vi "4.7.vi"() -> ()   [LabVIEW 2017]
panel:
  out "猜测次数":i32
  out "随机数":i32
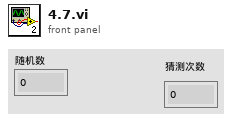
[diagram p1: front panel]
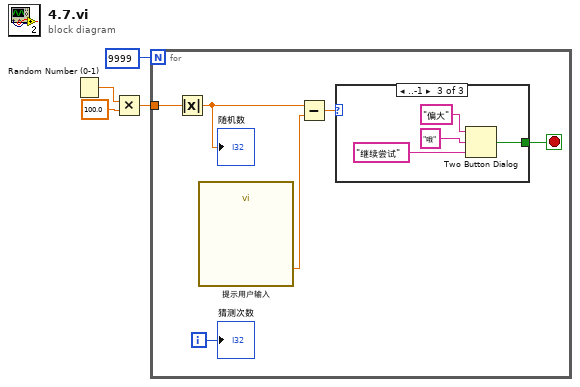
[diagram p0: block diagram]
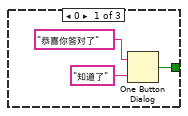
[diagram p2: hidden frame]
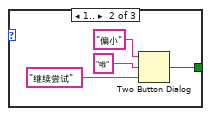
[diagram p3: hidden frame]
diagram:
  n1 = Random Number (0-1)() -> (number: 0 to 1=w2:dbl)
  n2 = Multiply(x=w2, y=100.0) -> (x*y=w3:dbl)
  n3 = for {
    N: 9999 -> [_]
    tunnel: w3 -> [w5]
    i -> [w8]
    stop <- w7 stop-if-true
    n4 = Absolute Value(x=w5) -> (abs(x)=w10:dbl)
    "随机数" <- w10
    n5 = call "提示用户输入"() -> ("请在1-1000猜"=w6:dbl)  [unwired: 17 in, 2 out]
    n6 = Subtract(x=w10, y=w6) -> (x-y=w9:dbl)
    n7 = case shown="..-1" w9 {
      tunnel: [w13 w14 w18] -> w7
      frame 0 {
        n8 = One Button Dialog(message="恭喜你答对了", button name ("OK")="知道了") -> (true=w13:bool)
      }
      frame 1.. {
        n9 = Two Button Dialog(message="偏小", 1:"继续尝试", 2:"哦") -> (T button?=w14:bool)
      }
      frame ..-1 {
        n10 = Two Button Dialog(message="偏大", 1:"继续尝试", 2:"哦") -> (T button?=w18:bool)
      }
    }
    "猜测次数" <- w8
  }
